vi "Teleop.vi"(10 "Match Info":T1={"Autonomous Elapsed Seconds"=0.0, "TeleOp Elapsed Seconds"=0.0, "Disabled Elapsed Seconds"=0.0, "Visited Autonomous"=FALSE, "Visited TeleOp"=FALSE, "Visited Disabled"=FALSE, "Autonomous Settings"={"Autonomous Style"=enum."Independent", "VI Refnum"=refnum}}, 11 "Call Context":T2) -> ()   [LabVIEW 2013]
doc: "This VI is called for each TeleOp packet received from the DS where the robot is not disabled. It is often used to read from the joysticks and update I/O or to update setpoints for timed control loops. It should complete and return within 20 milliseconds or it may miss DS packets."
uses:
  Robot Global Data.vi
  <vilib>/Rock Robotics/WPI/Solenoid/WPI_SolenoidSetEnum.vi
  <vilib>/Rock Robotics/WPI/Solenoid/WPI_SolenoidValue.ctl
  <vilib>/Rock Robotics/WPI/Solenoid/Deprecated/WPI_SolenoidGetBool.vi
  <vilib>/Rock Robotics/WPI/DriverStation/WPI_DriverStationMatch Info.ctl
  <vilib>/Rock Robotics/WPI/DriverStation/WPI_DriverStationDerivedRobotMode.ctl
panel:
  out "Numeric 1":dbl(slide) scale=0.0..100.0
  out "Boolean 2":bool
  out "Boolean 1":bool
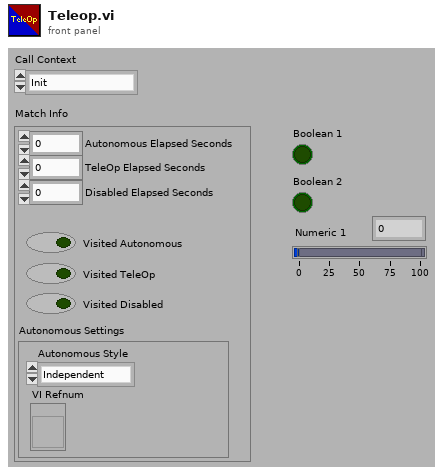
[diagram p1: front panel]
types:
  T1 = typedef "WPI_DriverStationMatch Info.ctl" = cluster{"Autonomous Elapsed Seconds":dbl, "TeleOp Elapsed Seconds":dbl, "Disabled Elapsed Seconds":dbl, "Visited Autonomous":bool, "Visited TeleOp":bool, "Visited Disabled":bool, "Autonomous Settings":cluster{"Autonomous Style":enum16{"Iterative", "Independent"}, "VI Refnum":refnum<vi>}}
  T2 = typedef "WPI_DriverStationDerivedRobotMode.ctl" = enum16{"Init", "Execute", "Stop"}
  T3 = typedef "WPI_SolenoidValue.ctl" = enum16{"Off", "On", "Forward", "Reverse"}
  T4 = typedef "WPI_JoystickDevRef.ctl" = cluster{"Device":T5}
  T5 = typedef "WPI_JoystickDeviceEnum.ctl" = enum16{"USB 1", "USB 2", "USB 3", "USB 4", "Kinect 1", "Kinect 2"}
  T6 = typedef "WPI_JoystickButtonState.ctl" = cluster{"Button 1":bool, "Button 2":bool, "Button 3":bool, "Button 4":bool, "Button 5":bool, "Button 6":bool, "Button 7":bool, "Button 8":bool, "Button 9":bool, "Button 10":bool, "Button 11":bool, "Button 12":bool}
  T7 = typedef "WPI_RobotDriveDevRef.ctl" = cluster{"DevStatus":errorcluster, "Motors[]":T8[], "Square Inputs":bool, "Max Output":dbl, "Isochronous":bool}
  T8 = typedef "WPI_MotorControlDeviceRef.ctl" = cluster{"DeviceStatus":errorcluster, "Type":enum16{"PWM", "CAN"}, "PWM":cluster{"Digital Module":T9, "PWM Channel":T10, "DeadBand":T11}, "CAN":cluster{"Device Number":u8, "Control Mode":T12, "Semaphore":T13, "Max Vout":dbl}, "Invert":bool, "TransformRef":T14, "InvTransformRef":T14}
  T9 = typedef "FPGA_TypedefDigitalModule.ctl" = enum16{"Digital Module 1", "Digital Module 2"}
  T10 = typedef "FPGA_DIOPWMChannel.ctl" = enum8{"PWM 1", "PWM 2", "PWM 3", "PWM 4", "PWM 5", "PWM 6", "PWM 7", "PWM 8", "PWM 9", "PWM 10", "Invalid"}
  T11 = typedef "WPI_PWMDeadband.ctl" = cluster{"Name":string, "maxPositivePwm":i32, "minPositivePwm":i32, "centerPwm":i32, "maxNegativePwm":i32, "minNegativePwm":i32, "angularRange":u16}
  T12 = typedef "WPI_CANJaguar_ControlMode.ctl" = enum8{"Percent VBus", "Current", "Speed", "Position", "Voltage"}
  T13 = typedef "Semaphore RefNum" = refnum<k1>
  T14 = typedef "WPI_PWMTransform_ConPane.ctl" = refnum<vi>
  T15 = cluster{"axis 1 (x)":dbl, "axis 2 (y)":dbl, "axis 3 (throttle)":dbl, "axis 4":dbl, "axis 5":dbl, "axis 6":dbl}
  T16 = typedef "WPI_AnalogChannelDevRef.ctl" = cluster{"DevStatus":errorcluster, "Analog Module":T17, "Analog Channel":T18}
  T17 = typedef "FPGA_TypedefAnalogModule.ctl" = enum16{"Analog Module 1", "Analog Module 2"}
  T18 = typedef "FPGA_AIChannel.ctl" = enum8{"AI 1", "AI 2", "AI 3", "AI 4", "AI 5", "AI 6", "AI 7", "AI 8", "Invalid"}
  T19 = typedef "WPI_RelayDevRef.ctl" = cluster{"DevStatus":errorcluster, "Relay Channel":T20, "Digital Module":T9, "Relay Direction":T21}
  T20 = typedef "FPGA_DIORelayChannel.ctl" = enum8{"Relay 1", "Relay 2", "Relay 3", "Relay 4", "Relay 5", "Relay 6", "Relay 7", "Relay 8", "Invalid"}
  T21 = typedef "WPI_RelayDirection.ctl" = enum16{"Both directions", "Forward only", "Reverse only"}
  T22 = typedef "WPI_SolenoidDevRef.ctl" = cluster{"DevStatus":errorcluster, "Solenoid Module":T23, "Forward Solenoid Channel":T24, "Reverse Solenoid Channel":T24}
  T23 = typedef "FPGA_TypedefSolenoidModule.ctl" = enum16{"Solenoid Module 1", "Solenoid Module 2"}
  T24 = typedef "WPI_SolenoidChannel.ctl" = enum8{"Solenoid 1", "Solenoid 2", "Solenoid 3", "Solenoid 4", "Solenoid 5", "Solenoid 6", "Solenoid 7", "Solenoid 8", "Invalid"}
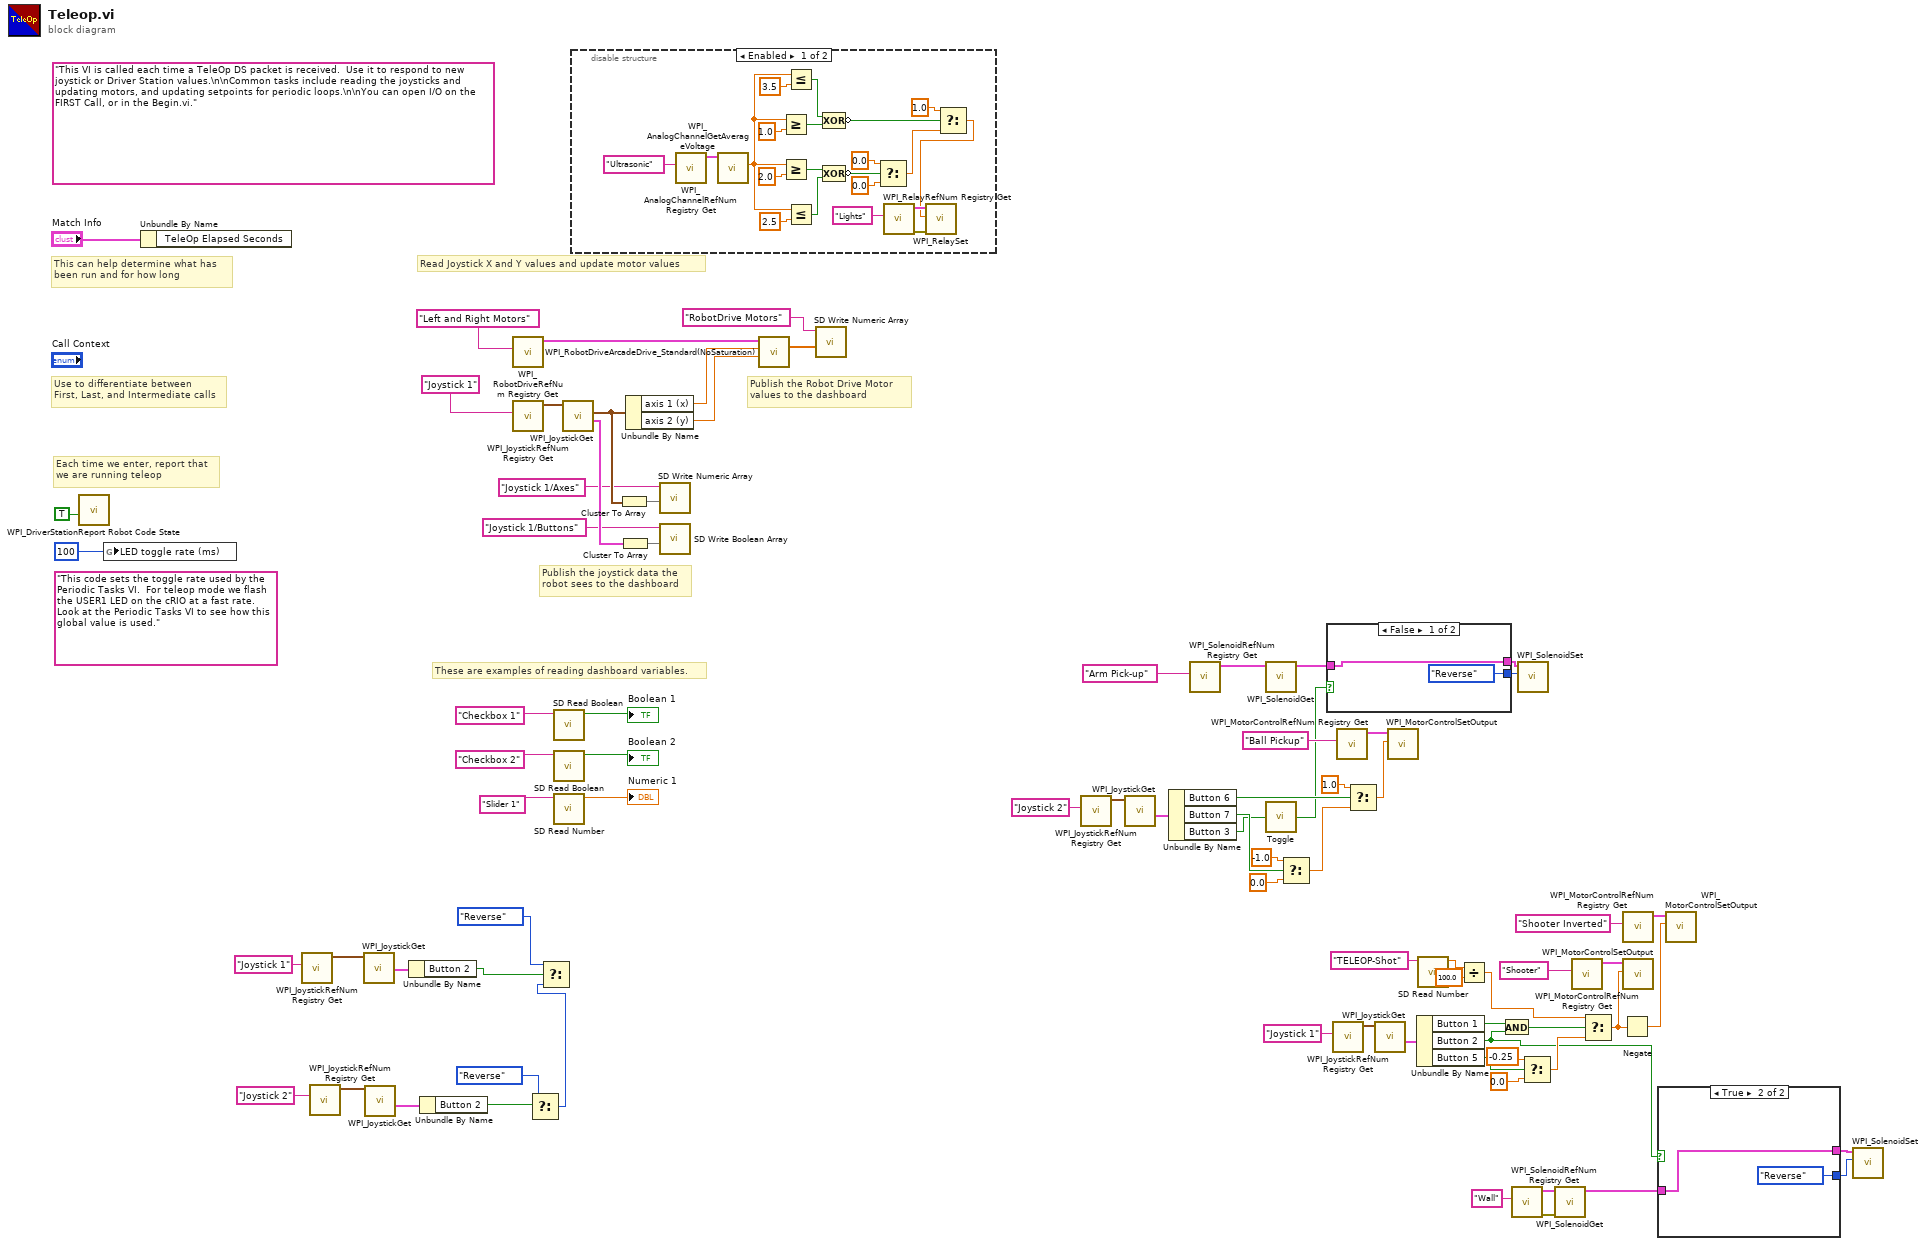
[diagram p0: block diagram]
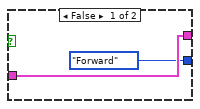
[diagram p2: hidden frame]
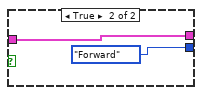
[diagram p4: hidden frame]
diagram:
  (unwired) "This code sets the toggle rate used by the Periodic Tasks VI.  For teleop mode we flash the USER1 LED on the cRIO at a fast rate.  Look at the Periodic Tasks VI to see how this global value is used."
  (unwired) "This VI is called each time a TeleOp DS packet is received.  Use it to respond to new joystick or Driver Station values.\n\nCommon tasks include reading the joysticks and updating motors, and updating setpoints for periodic loops.\n\nYou can open I/O on the FIRST Call, or in the Begin.vi."
  # "These are examples of reading dashboard variables."
  # "Publish the Robot Drive Motor\nvalues to the dashboard"
  # "Publish the joystick data the\nrobot sees to the dashboard"
  # "Each time we enter, report that\nwe are running teleop"
  # "Use to differentiate between\nFirst, Last, and Intermediate calls"
  # "This can help determine what has\nbeen run and for how long"
  # "Read Joystick X and Y values and update motor values"
  n1 = call <vilib>:"WPI_DriverStationReport Robot Code State.vi"("TeleOp"=TRUE ("Autonomous")) -> ()  [unwired: 10 in, 1 out]
  n2 = global write "Robot Global Data.vi" "LED toggle rate (ms)"(u32 100 ("LED ms toggle rate")) -> ()
  n3 = Unbundle By Name("Match Info") -> ()  [unwired: 1 out]
  n4 = call <vilib>:"WPI_JoystickRefNum Registry Get.vi"("refnum name"="Joystick 1") -> ("JoystickDevRef"=w8:T4)  [unwired: 9 in, 1 out]
  n5 = call <vilib>:"WPI_JoystickRefNum Registry Get.vi"("refnum name"="Joystick 2") -> ("JoystickDevRef"=w9:T4)  [unwired: 9 in, 1 out]
  n6 = call <vilib>:"WPI_JoystickGet.vi"("JoystickDevRef"=w8) -> ("Buttons"=w7:T6)  [unwired: 4 in, 2 out]
  n7 = call <vilib>:"WPI_JoystickGet.vi"("JoystickDevRef"=w9) -> ("Buttons"=w6:T6)  [unwired: 4 in, 2 out]
  n8 = Unbundle By Name(w7) -> ("Button 2"=w5:bool)
  n9 = Unbundle By Name(w6) -> ("Button 2"=w4:bool)
  n10 = call <vilib>:"WPI_RobotDriveRefNum Registry Get.vi"("refnum name"="Left and Right Motors") -> ("RobotDriveDevRef"=w77:T7)  [unwired: 1 in, 9 out]
  n11 = call <vilib>:"WPI_JoystickRefNum Registry Get.vi"("refnum name"="Joystick 1") -> ("JoystickDevRef"=w73:T4)  [unwired: 1 in, 9 out]
  n12 = Select(t=WPI_SolenoidValue."Reverse" ("Value"), s=w4) -> (s? t:f=w1:T3)  [unwired: 1 in]
  n13 = Select(t=WPI_SolenoidValue."Reverse" ("Value"), s=w5, f=w1) -> ()  [unwired: 1 out]
  n14 = call <vilib>:"SD Read Boolean.vi"("Name"="Checkbox 1" ("refnum name")) -> ("Boolean"=→"Boolean 1":bool)  [unwired: 8 in, 2 out]
  n15 = call <vilib>:"SD Read Boolean.vi"("Name"="Checkbox 2" ("refnum name")) -> ("Boolean"=→"Boolean 2":bool)  [unwired: 8 in, 2 out]
  n16 = call <vilib>:"SD Read Number.vi"("Name"="Slider 1" ("refnum name")) -> ("Numeric"=→"Numeric 1":dbl)  [unwired: 8 in, 2 out]
  n17 = call <vilib>:"WPI_JoystickGet.vi"("JoystickDevRef"=w73) -> ("Buttons"=w70:T6, "Axes"=w67:T15)  [unwired: 1 in, 4 out]
  n18 = disable-structure shown="Enabled" {
    frame Enabled {
      n19 = call <vilib>:"WPI_AnalogChannelRefNum Registry Get.vi"("refnum name"="Ultrasonic") -> ("AIDeviceRef"=w99:T16)  [unwired: 9 in, 1 out]
      n20 = call <vilib>:"WPI_AnalogChannelGetAverageVoltage.vi"("AIDeviceRef"=w99) -> ("Voltage"=w90:dbl)  [unwired: 8 in, 2 out]
      n21 = Greater Or Equal?(x=w90, y=1.0) -> (x >= y?=w93:bool)
      n22 = Greater Or Equal?(x=w90, y=2.0) -> (x >= y?=w87:bool)
      n23 = Less Or Equal?(x=w90, y=3.5) -> (x <= y?=w92:bool)
      n24 = Less Or Equal?(x=w90, y=2.5) -> (x <= y?=w88:bool)
      n25 = Compound Arithmetic op=XOR(w92, w93) -> (invert w85:bool)
      n26 = Compound Arithmetic op=XOR(w87, w88) -> (invert w86:bool)
      n27 = Select(t=0.0, s=w86, f=0.0) -> (s? t:f=w81:dbl)
      n28 = call <vilib>:"WPI_RelayRefNum Registry Get.vi"("refnum name"="Lights") -> ("error out"=w98:errorcluster, "RelayDevRef"=w97:T19)  [unwired: 9 in]
      n29 = Select(t=1.0, s=w85, f=w81) -> (s? t:f=w80:dbl)
      n30 = call <vilib>:"WPI_RelaySet.vi"("error in (no error)"=w98, "RelayValue"=w80, "RelayDevRef"=w97) -> ()  [unwired: 7 in, 2 out]
    }
    frame Disabled {
    }
  }
  n31 = Cluster To Array(cluster=w67) -> (array=w66:dbl[])
  n32 = Cluster To Array(cluster=w70) -> (array=w69:bool[])
  n33 = Unbundle By Name(w67) -> ("axis 1 (x)"=w76:dbl, "axis 2 (y)"=w75:dbl)
  n34 = call <vilib>:"SD Write Numeric Array.vi"("Numeric Array"=w66, "Name"="Joystick 1/Axes") -> ()  [unwired: 8 in, 2 out]
  n35 = call <vilib>:"SD Write Boolean Array.vi"("Boolean Array"=w69, "Name"="Joystick 1/Buttons") -> ()  [unwired: 8 in, 2 out]
  n36 = call <vilib>:"WPI_RobotDriveArcadeDrive_Standard(NoSaturation).vi"("Y axis value"=w75, "X axis value"=w76, "RobotDriveDevRef"=w77) -> ("Motor Values"=w63:dbl[])  [unwired: 1 in, 7 out]
  n37 = call <vilib>:"SD Write Numeric Array.vi"("Numeric Array"=w63, "Name"="RobotDrive Motors") -> ()  [unwired: 8 in, 2 out]
  n38 = call <vilib>:"WPI_JoystickRefNum Registry Get.vi"("refnum name"="Joystick 2") -> ("JoystickDevRef"=w41:T4)  [unwired: 1 in, 9 out]
  n39 = call <vilib>:"WPI_JoystickGet.vi"("JoystickDevRef"=w41) -> ("Buttons"=w39:T6)  [unwired: 1 in, 5 out]
  n40 = Unbundle By Name(w39) -> ("Button 6"=w37:bool, "Button 7"=w38:bool, "Button 3"=w29:bool)
  n41 = call <vilib>:"WPI_SolenoidRefNum Registry Get.vi"("refnum name"="Arm Pick-up") -> ("SolenoidDevRef"=w27:T22)  [unwired: 9 in, 1 out]
  n42 = call-poly <vilib>:"WPI_SolenoidGet.vi"("SolenoidDevRef"=w27) -> ("SolenoidDevRef"=w26:T22)  [unwired: 8 in, 2 out]
  n43 = call "Toggle.vi"("Input"=w29) -> ("Toggled Output"=w28:bool)
  n44 = Select(t=-1.0, s=w38, f=0.0) -> (s? t:f=w33:dbl)
  n45 = case shown="False" w28 {
    tunnel: w26 -> [w102 w104]
    tunnel: [w102 w104] -> w22
    tunnel: [WPI_SolenoidValue."Reverse" ("Value") WPI_SolenoidValue."Forward" ("Value")] -> w21
    frame False {
    }
    frame True {
    }
  }
  n46 = call <vilib>:"WPI_JoystickRefNum Registry Get.vi"("refnum name"="Joystick 1") -> ("JoystickDevRef"=w55:T4)  [unwired: 1 in, 9 out]
  n47 = call <vilib>:"WPI_MotorControlRefNum Registry Get.vi"("refnum name"="Ball Pickup") -> ("MotorControlDevRef"=w31:T8)  [unwired: 9 in, 1 out]
  n48 = Select(t=1.0, s=w37, f=w33) -> (s? t:f=w30:dbl)
  n49 = call <vilib>:"WPI_JoystickGet.vi"("JoystickDevRef"=w55) -> ("Buttons"=w54:T6)  [unwired: 1 in, 5 out]
  n50 = call <vilib>:"WPI_MotorControlSetOutput.vi"("Output"=w30, "MotorControlDevRef"=w31) -> ()  [unwired: 7 in, 3 out]
  n51 = Unbundle By Name(w54) -> ("Button 1"=w53:bool, "Button 2"=w16:bool, "Button 5"=w51:bool)
  n52 = call <vilib>:"SD Read Number.vi"("Name"="TELEOP-Shot") -> ("Numeric"=w14:dbl)  [unwired: 8 in, 2 out]
  n53 = Divide(x=w14, y=100.0) -> (x/y=w12:dbl)
  n54 = And(x=w53, y=w16) -> (x .and. y?=w52:bool)
  n55 = call <vilib>:"WPI_SolenoidRefNum Registry Get.vi"("refnum name"="Wall") -> ("error out"=w24:errorcluster, "SolenoidDevRef"=w23:T22)  [unwired: 9 in]
  n56 = call-poly <vilib>:"WPI_SolenoidSet.vi"("Value"=w21, "SolenoidDevRef"=w22) -> ()  [unwired: 8 in, 2 out]
  n57 = Select(t=-0.25, s=w51, f=0.0) -> (s? t:f=w48:dbl)
  n58 = call-poly <vilib>:"WPI_SolenoidGet.vi"("error in (no error)"=w24, "SolenoidDevRef"=w23) -> ("SolenoidDevRef"=w20:T22)  [unwired: 7 in, 2 out]
  n59 = call <vilib>:"WPI_MotorControlRefNum Registry Get.vi"("refnum name"="Shooter") -> ("MotorControlDevRef"=w46:T8)  [unwired: 9 in, 1 out]
  n60 = Select(t=w12, s=w52, f=w48) -> (s? t:f=w45:dbl)
  n61 = Negate(x=w45) -> (-x=w43:dbl)
  n62 = call <vilib>:"WPI_MotorControlRefNum Registry Get.vi"("refnum name"="Shooter Inverted") -> ("MotorControlDevRef"=w42:T8)  [unwired: 9 in, 1 out]
  n63 = call <vilib>:"WPI_MotorControlSetOutput.vi"("Output"=w45, "MotorControlDevRef"=w46) -> ()  [unwired: 7 in, 3 out]
  n64 = case shown="True" w16 {
    tunnel: w20 -> [w106 w108]
    tunnel: [w106 w108] -> w19
    tunnel: [WPI_SolenoidValue."Forward" ("Value") WPI_SolenoidValue."Reverse" ("Value")] -> w18
    frame False {
    }
    frame True {
    }
  }
  n65 = call <vilib>:"WPI_MotorControlSetOutput.vi"("Output"=w43, "MotorControlDevRef"=w42) -> ()  [unwired: 7 in, 3 out]
  n66 = call-poly <vilib>:"WPI_SolenoidSet.vi"("Value"=w18, "SolenoidDevRef"=w19) -> ()  [unwired: 8 in, 2 out]
